vi "CTRE_Phoenix_CANdle_SetLEDs.vi"(0 "CTRE_CANdle_DeviceRef":T2, 5 "Start Index":i32, 7 "Count":i32=512, 9 "LED Color":T1, 11 "error in":errorcluster) -> (4 "CTRE_CANdle_DeviceRef":T2, 15 "error out":errorcluster)   [LabVIEW 2020]
doc: "Sets a contiguous block of LEDs to the specified color. <b>Start Index</b> and <b>Count</b> default to values that will set all LEDs to the specified color.\n\n<b>Start Index</b> is the index of the first LED in the block to be set. LEDs are zero-indexed starting with LEDs 0 through 7 onboard the CANdle. LED 8 is the first LED of an external strip.\n\n<b>Count</b> is the number of LEDs to set including the LED at the <b>Start Index</b>.\n\n<b>LED Color</b> is the cluster of RGBW values that define the color of the LED block. White is only used if the LED strip type supports a white element."
uses:
  <vilib>/Rock Robotics/WPI/ThirdParty/Phoenix-LabVIEW/CANdle/Controls/CTRE_Phoenix_CANdle_DeviceRef.ctl
  <vilib>/Rock Robotics/WPI/ThirdParty/Phoenix-LabVIEW/CANdle/Controls/CTRE_Phoenix_CANdle_LEDColor.ctl
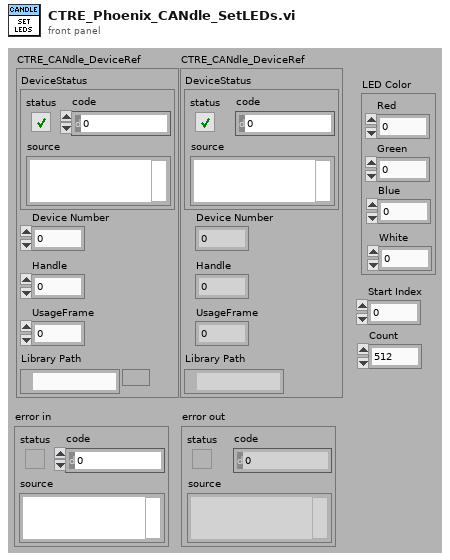
[diagram p1: front panel]
types:
  T1 = typedef "CTRE_Phoenix_CANdle_LEDColor.ctl" = cluster{"Red":u8, "Green":u8, "Blue":u8, "White":u8}
  T2 = typedef "CTRE_Phoenix_CANdle_DeviceRef.ctl" = cluster{"DeviceStatus":errorcluster, "Device Number":u8, "Handle":u64, "UsageFrame":u32, "Library Path":path}
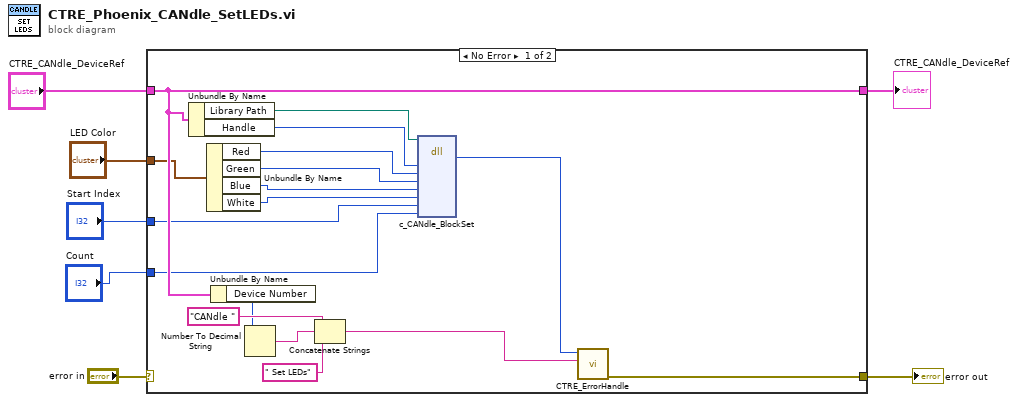
[diagram p0: block diagram]
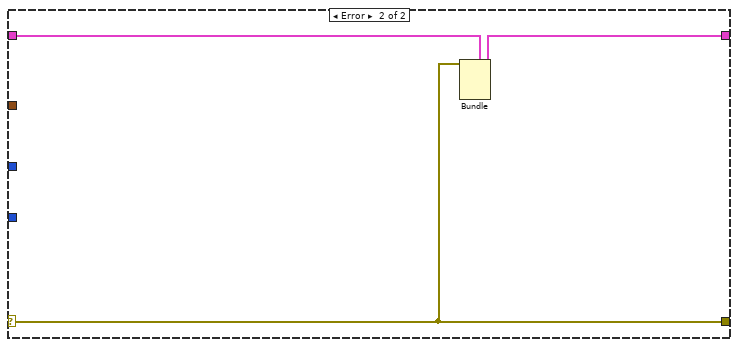
[diagram p2: hidden frame]
diagram:
  n1 = case shown="No Error" "error in" {
    selector: "error in" -> [_ w26]
    tunnel: "CTRE_CANdle_DeviceRef" -> [w17 w27]
    tunnel: [w24 w26] -> w7
    tunnel: [w17 w25] -> w4
    tunnel: "LED Color" -> [w14 _]
    tunnel: "Start Index" -> [w9 _]
    tunnel: "Count" -> [w8 _]
    frame No Error {
      n2 = Unbundle By Name(w17) -> ("Library Path"=w16:path, "Handle"=w15:u64)
      n3 = Unbundle By Name(w14) -> ("Red"=w13:u8, "Green"=w12:u8, "Blue"=w11:u8, "White"=w10:u8)
      n4 = Unbundle By Name(w17) -> ("Device Number"=w20:u8)
      n5 = Number To Decimal String(number=w20) -> (decimal integer string=w22:string)  [unwired: 1 in]
      n6 = Concatenate Strings("CANdle " ("string"), w22, " Set LEDs" ("string")) -> (w18:string)
      n7 = dll-call lib="?" fn="c_CANdle_BlockSet"(path in=w16, "handle"=w15, "r"=w13, "g"=w12, "b"=w11, "w"=w10, "startIdx"=w9, "count"=w8) -> ("return type"=w19:i32)  [unwired: 9 in, 2 out]
      n8 = call <vilib>:"CTRE_ErrorHandle.vi"("origin"=w18, "code"=w19) -> ("error out"=w24:errorcluster)  [unwired: 9 in]
    }
    frame Error {
      n9 = Bundle(cluster=w27, "DeviceStatus"=w26) -> (w25:T2)  [unwired: 4 in]
    }
  }
  "error out" <- w7
  "CTRE_CANdle_DeviceRef" <- w4
